vi "Char en archivo txt.vi"() -> ()   [LabVIEW 2010]
panel:
  in  "stop":bool
  out "Waveform Chart":dbl(graph)
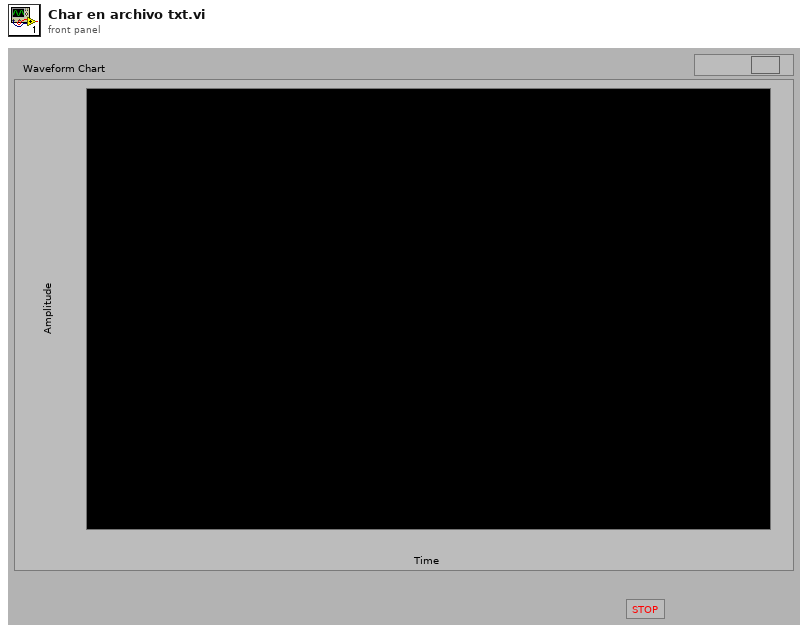
[diagram p1: front panel]
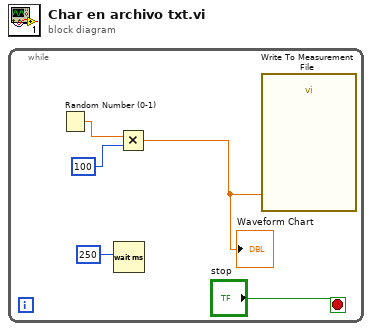
[diagram p0: block diagram]
diagram:
  n1 = while {
    stop <- "stop" stop-if-true
    n2 = Random Number (0-1)() -> (number: 0 to 1=w5:dbl)
    n3 = Wait (ms)(milliseconds to wait=250) -> ()  [unwired: 1 out]
    n4 = Multiply(x=w5, y=100) -> (x*y=w1:dbl)
    "Waveform Chart" <- w1
    n5 = call "Write To Measurement File"("Signals"=w1) -> ()  [unwired: 16 in, 3 out]
  }
